vi "Begin.vi"(8 "error in":errorcluster) -> (0 "error out":errorcluster)   [LabVIEW 2019]
doc: "Called before other user functions, this VI is expected to open initial I/O refnums, load in file data, and do all program initialization. Notice that the <B>error out</B> terminal is simply used for data flow. Wiring it to other structures or subVIs ensures that this VI runs first."
uses:
  <vilib>/Rock Robotics/WPI/DriverStation/WPI_DriverStationRobotMode2.ctl
  Subsystems/Drive/Drive_Cluster.ctl
  Subsystems/Drive/Drive_States.ctl
  Subsystems/Intake/Intake_Cluster.ctl
  Subsystems/Intake/Intake_States.ctl
  Subsystems/Turret/Turret_Cluster.ctl
  Subsystems/Turret/Turret_States.ctl
  Subsystems/Magazine/Magazine_Cluster.ctl
  Subsystems/Magazine/Magazine_States.ctl
  Subsystems/Climb/Climb_Cluster.ctl
  Subsystems/Climb/Climb_States.ctl
  Subsystems/Control_Panel/Control_Panel_Cluster.ctl
  Subsystems/Control_Panel/Control_Panel_States.ctl
  <vilib>/Rock Robotics/WPI/Joystick/WPI_JoystickDeviceEnum.ctl
  <vilib>/Rock Robotics/WPI/ThirdParty/REV Robotics/SPARK MAX/Typedef/Spark MAX Control Type.ctl
  Subsystems/Flywheel/Flywheel_Cluster.ctl
  Subsystems/Flywheel/Flywheel_States.ctl
  <vilib>/Rock Robotics/WPI/ThirdParty/Phoenix-LabVIEW/Motor Controller/Controls/CTRE_Phoenix_MotorControl_ControlMode.ctl
  <vilib>/Rock Robotics/WPI/ThirdParty/REV Robotics/SPARK MAX/Typedef/Spark MAX Idle Mode.ctl
  <vilib>/Rock Robotics/WPI/ThirdParty/REV Robotics/SPARK MAX/Typedef/Spark MAX Motor Type.ctl
  <vilib>/Rock Robotics/WPI/ThirdParty/Phoenix-LabVIEW/Motor Controller/Controls/CTRE_Phoenix_MotorControl_SupplyCurrentLimitConfiguration.ctl
  Robot Global Data.vi
  Globals/Drive_Globals.vi
  Globals/Intake_Globals.vi
  Globals/Turret_Globals.vi
  Globals/Magazine_Globals.vi
  Globals/Climb_Globals.vi
  Globals/Control_Panel_Globals.vi
  Globals/Joystick_Globals.vi
  Globals/Flywheel_Globals.vi
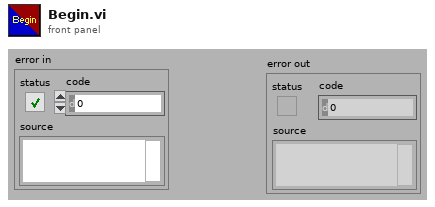
[diagram p1: front panel]
types:
  T1 = typedef "CTRE_Phoenix_MotorControl_SupplyCurrentLimitConfiguration.ctl" = cluster{"Enable?":bool, "Current Limit":dbl, "Threshold Current":dbl, "Threshold Time":dbl}
  T2 = typedef "Spark MAX Idle Mode.ctl" = enum16{"Coast", "Brake"}
  T3 = typedef "Spark MAX Motor Type.ctl" = enum16{"Brushed", "Brushless"}
  T4 = typedef "CTRE_Phoenix_MotorControl_ControlMode.ctl" = u16
  T5 = typedef "Spark MAX Control Type.ctl" = enum16{"Percent VBus", "Voltage", "Velocity", "Position", "Smart Motion", "Current", "Smart Velocity"}
  T6 = cluster{"P Gain":dbl, "I Gain":dbl, "D Gain":dbl, "F Gain":dbl, "I Zone":dbl, "Min Output":dbl, "Max Output":dbl}
  T7 = typedef "Flywheel_Cluster.ctl" = cluster{"Flywheel_Throttle":dbl, "Control_States":T8, "Auto_Speed":bool, "Flywheel_On":bool}
  T8 = typedef "Flywheel_States.ctl" = enum16{"No-Op", "Percent_Voltage", "Speed_Control_Manual", "Speed_Control_Auto"}
  T9 = typedef "WPI_JoystickDeviceEnum.ctl" = enum16{"USB 0", "USB 1", "USB 2", "USB 3", "USB 4", "USB 5"}
  T10 = typedef "Control_Panel_Cluster.ctl" = cluster{"Control_State":T11, "Start_Movement":bool, "Abort":bool, "Rotation_Control?":bool, "Positional_Control? ":bool, "Throttle":dbl}
  T11 = typedef "Control_Panel_States.ctl" = enum16{"No-Op", "Rotational_Control", "Positional_Control", "Manual_Control"}
  T12 = typedef "Climb_Cluster.ctl" = cluster{"Control_State":T13, "Extend_Climber?":bool, "Clamp?":bool, "Balance?":bool, "Transverse_Throttle":dbl, "Elevator_Throttle":dbl, "Control_Panel_Setpoint?":bool, "Auto-Balance":bool, "Pivot_Throttle":dbl}
  T13 = typedef "Climb_States.ctl" = enum16{"No-Op", "Extending", "Clamping", "Balancing", "Manual_Control"}
  T14 = typedef "Magazine_Cluster.ctl" = cluster{"Control_States":T15, "Fire":bool, "Magazine_Throttle":dbl}
  T15 = typedef "Magazine_States.ctl" = enum16{"No-Op", "Loading", "Fire", "Unjam", "Manual"}
  T16 = typedef "Turret_Cluster.ctl" = cluster{"Auto-Target?":bool, "Control_State":T17, "Turret_Spin_Speed":dbl, "Turret_Spin_Speed_Control?":bool}
  T17 = typedef "Turret_States.ctl" = enum16{"Manual_Percent_Voltage", "Manual_Speed_Control", "Auto-Target"}
  T18 = typedef "Intake_Cluster.ctl" = cluster{"Control_State":T19, "Intake_On":bool, "Intake_Extended":bool, "Intake_Throttle":dbl}
  T19 = typedef "Intake_States.ctl" = enum16{"Manual_Control"}
  T20 = typedef "Drive_Cluster.ctl" = cluster{"Control_State":T21, "Angular_Throttle":dbl, "Linear_Throttle":dbl, "Torque_Changing":bool}
  T21 = typedef "Drive_States.ctl" = enum16{"Percent_Voltage_Control", "Speed_Control"}
  T22 = typedef "WPI_DriverStationRobotMode2.ctl" = enum16{"Autonomous Disabled", "Autonomous Enabled", "Teleop Disabled", "Teleop Enabled", "Disconnected", "Finish", "Test Disabled", "Test Enabled", "Emergency Stopped"}
  T23 = typedef "WPI_JoystickDevRef.ctl" = cluster{"Device":T9}
  T24 = typedef "WPI_MotorControlDeviceRef.ctl" = cluster{"DeviceStatus":errorcluster, "Type":T25, "PWM":cluster{"PWM Channel":T26, "DeadBand":T27}, "CAN":cluster{"Device Number":u8, "SetOutput VI Ref":variant, "GetOutput VI Ref":variant, "Enable VI Ref":variant, "Disable VI Ref":variant, "Data":variant}, "Invert":bool, "DIO PWM":cluster{"PWM \"Enable\" Channel":T26, "DIOChannel":T28, "PWM Rate":dbl}}
  T25 = typedef "WPI_MotorControlType.ctl" = enum16{"PWM", "CAN", "DIO PWM"}
  T26 = typedef "FPGA_DIOPWMChannel.ctl" = enum8{"PWM 0", "PWM 1", "PWM 2", "PWM 3", "PWM 4", "PWM 5", "PWM 6", "PWM 7", "PWM 8", "PWM 9", "PWM MXP 0", "PWM MXP 1", "PWM MXP 2", "PWM MXP 3", "PWM MXP 4", "PWM MXP 5", "PWM MXP 6", "PWM MXP 7", "PWM MXP 8", "PWM MXP 9", "Invalid"}
  T27 = typedef "WPI_PWMDeadband.ctl" = cluster{"Name":string, "maxPositivePwm":i32, "minPositivePwm":i32, "centerPwm":i32, "maxNegativePwm":i32, "minNegativePwm":i32, "angularRange":u16}
  T28 = typedef "FPGA_DIOChannel.ctl" = enum8{"DIO 0", "DIO 1", "DIO 2", "DIO 3", "DIO 4", "DIO 5", "DIO 6", "DIO 7", "DIO 8", "DIO 9", "DIO MXP 0", "DIO MXP 1", "DIO MXP 2", "DIO MXP 3", "DIO MXP 4", "DIO MXP 5", "DIO MXP 6", "DIO MXP 7", "DIO MXP 8", "DIO MXP 9", "DIO MXP 10", "DIO MXP 11", "DIO MXP 12", "DIO MXP 13", "DIO MXP 14", "DIO MXP 15", "SPI Port CS1", "SPI Port CS2", "SPI Port CS3", "SPI Port MISO", "SPI Port MOSI", "Invalid"}
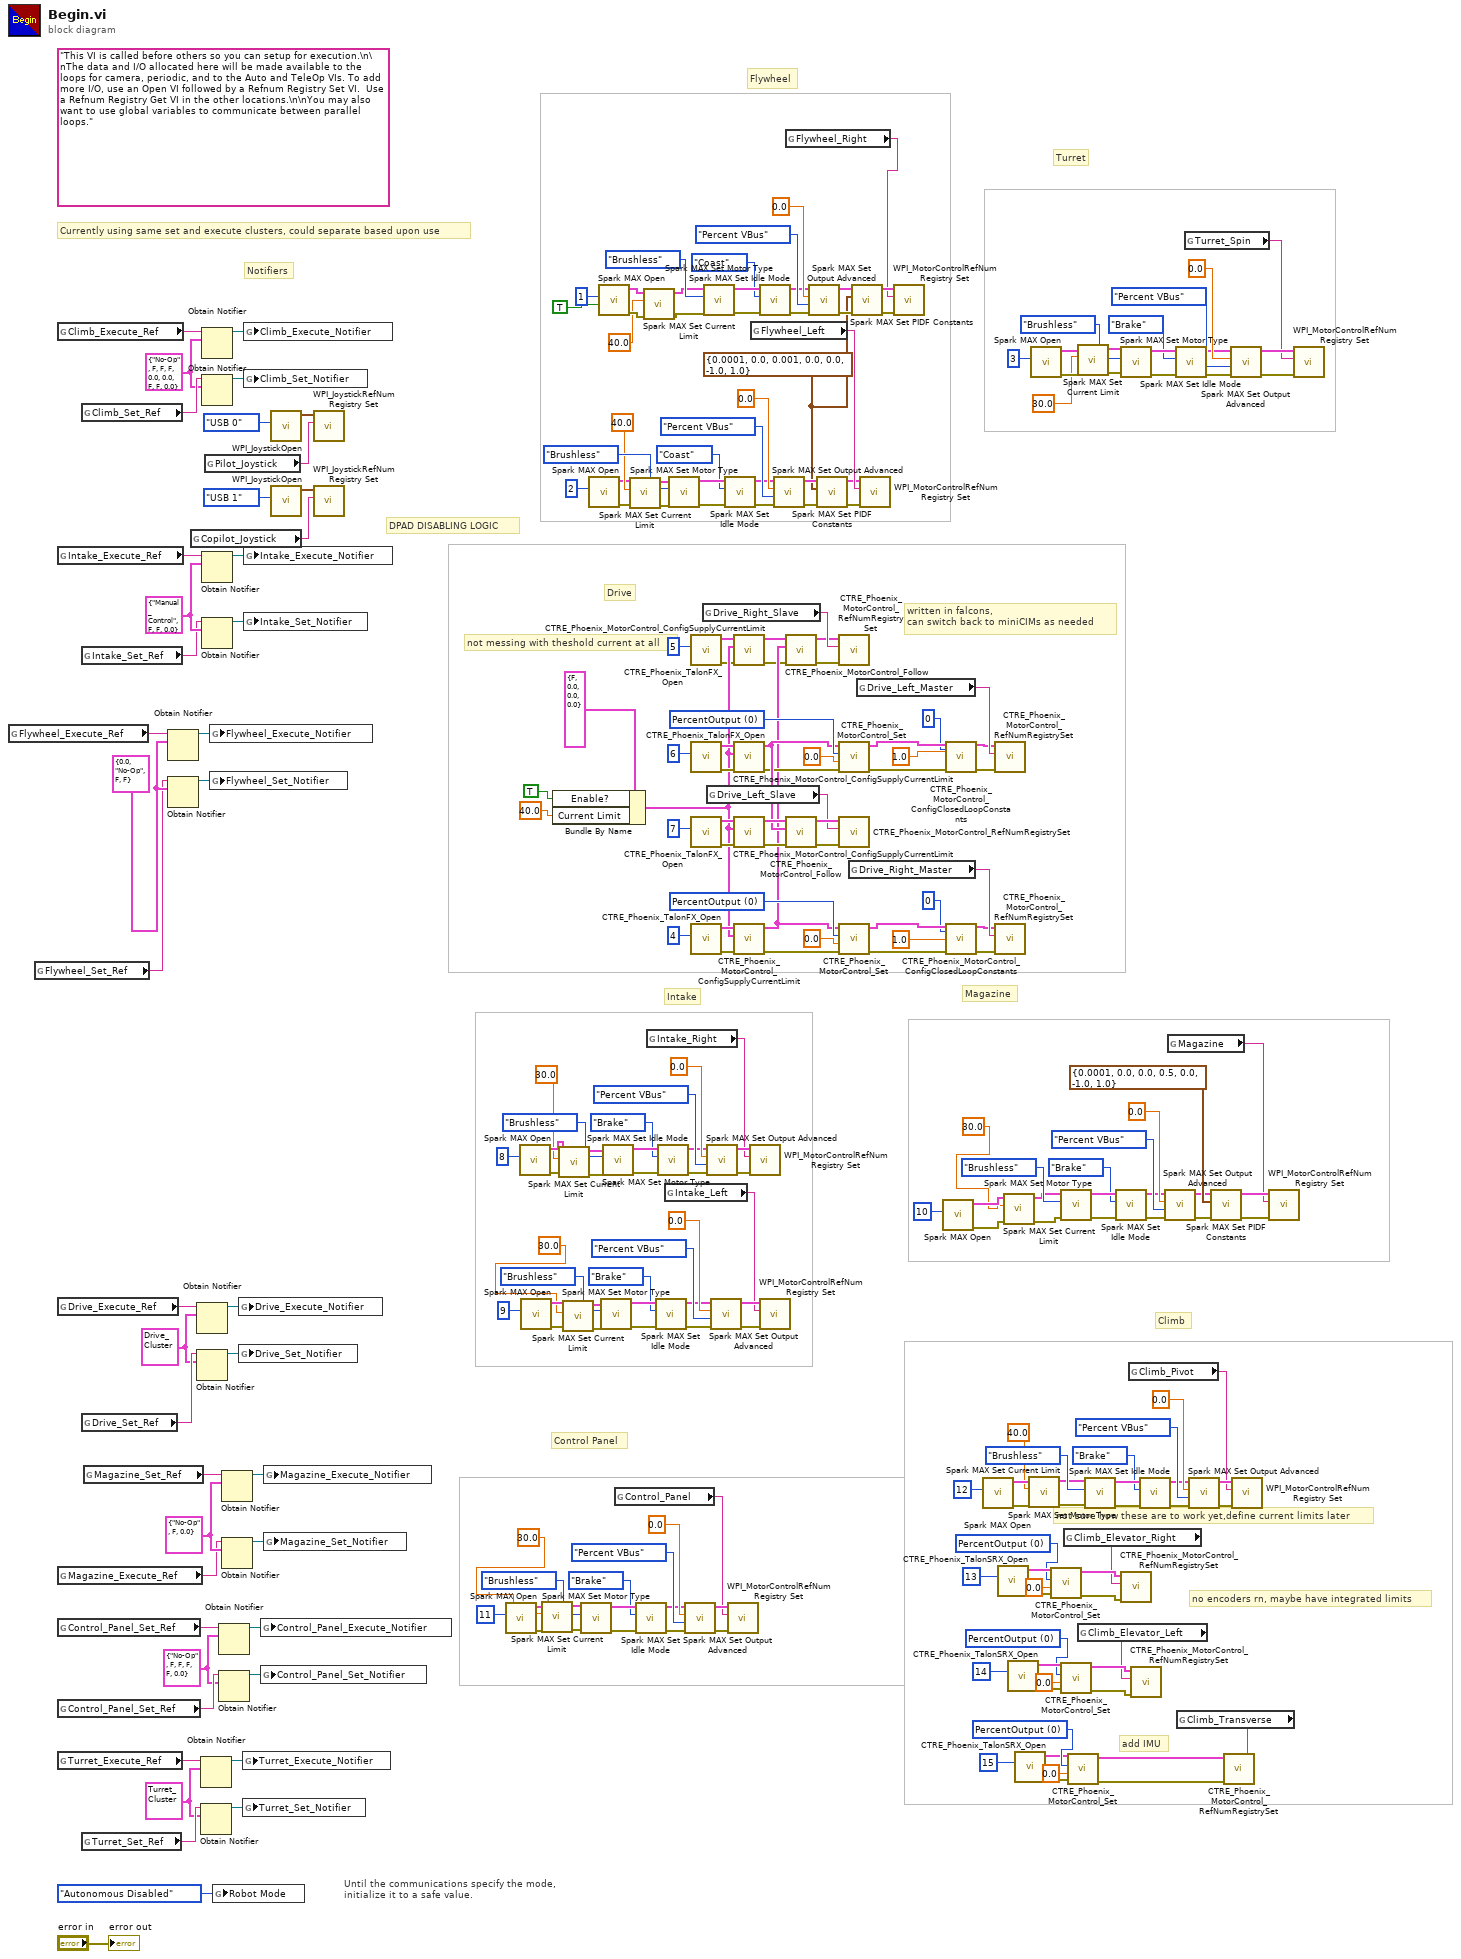
[diagram p0: block diagram]
diagram:
  w119 = T4 0 items=["PercentOutput"=0, "Position"=1, "Velocity"=2, "Current"=3, "Follower"=5, "MotionProfile"=6, "MotionMagic"=7, "MotionProfileArc"=10, "Disabled"=15] ("Control Mode")
  w126 = T4 0 items=["PercentOutput"=0, "Position"=1, "Velocity"=2, "Current"=3, "Follower"=5, "MotionProfile"=6, "MotionMagic"=7, "MotionProfileArc"=10, "Disabled"=15] ("Control Mode")
  w135 = T4 0 items=["PercentOutput"=0, "Position"=1, "Velocity"=2, "Current"=3, "Follower"=5, "MotionProfile"=6, "MotionMagic"=7, "MotionProfileArc"=10, "Disabled"=15] ("Control Mode")
  w168 = T7 {"Flywheel_Throttle"=0.0, "Control_States"=enum."No-Op", "Auto_Speed"=FALSE, "Flywheel_On"=FALSE}
  w1 = T6 {"P Gain"=0.0001, "I Gain"=0.0, "D Gain"=0.001, "F Gain"=0.0, "I Zone"=0.0, "Min Output"=-1.0, "Max Output"=1.0} ("PID Constants")
  w207 = T4 0 items=["PercentOutput"=0, "Position"=1, "Velocity"=2, "Current"=3, "Follower"=5, "MotionProfile"=6, "MotionMagic"=7, "MotionProfileArc"=10, "Disabled"=15] ("Control Mode")
  w217 = T4 0 items=["PercentOutput"=0, "Position"=1, "Velocity"=2, "Current"=3, "Follower"=5, "MotionProfile"=6, "MotionMagic"=7, "MotionProfileArc"=10, "Disabled"=15] ("Control Mode")
  w241 = T10 {"Control_State"=enum."No-Op", "Start_Movement"=FALSE, "Abort"=FALSE, "Rotation_Control?"=FALSE, "Positional_Control? "=FALSE, "Throttle"=0.0}
  w245 = T12 {"Control_State"=enum."No-Op", "Extend_Climber?"=FALSE, "Clamp?"=FALSE, "Balance?"=FALSE, "Transverse_Throttle"=0.0, "Elevator_Throttle"=0.0, "Control_Panel_Setpoint?"=FALSE, "Auto-Balance"=FALSE, "Pivot_Throttle"=0.0}
  w249 = T14 {"Control_States"=enum."No-Op", "Fire"=FALSE, "Magazine_Throttle"=0.0}
  w250 = T16 {"Auto-Target?"=FALSE, "Control_State"=enum."Manual_Percent_Voltage", "Turret_Spin_Speed"=0.0, "Turret_Spin_Speed_Control?"=FALSE}
  w255 = T18 {"Control_State"=enum."Manual_Control", "Intake_On"=FALSE, "Intake_Extended"=FALSE, "Intake_Throttle"=0.0}
  w256 = T20 {"Control_State"=enum."Percent_Voltage_Control", "Angular_Throttle"=0.0, "Linear_Throttle"=0.0, "Torque_Changing"=FALSE}
  (unwired) "This VI is called before others so you can setup for execution.\n\nThe data and I/O allocated here will be made available to the loops for camera, periodic, and to the Auto and TeleOp VIs. To add more I/O, use an Open VI followed by a Refnum Registry Set VI.  Use a Refnum Registry Get VI in the other locations.\n\nYou may also want to use global variables to communicate between parallel loops."
  # "not sure how these are to work yet,define current limits later"
  # "not messing with theshold current at all"
  # "add IMU"
  # "no encoders rn, maybe have integrated limits"
  # "Climb"
  # "Control Panel"
  # "Magazine"
  # "Intake"
  # "written in falcons, \ncan switch back to miniCIMs as needed"
  # "Drive"
  # "Turret"
  # "Flywheel"
  # "DPAD DISABLING LOGIC"
  # "Notifiers"
  # "Currently using same set and execute clusters, could separate based upon use"
  # "Until the communications specify the mode,\ninitialize it to a safe value."
  n1 = global read "Flywheel_Globals.vi" "Flywheel_Execute_Ref"() -> (w167:string)
  n2 = global read "Flywheel_Globals.vi" "Flywheel_Set_Ref"() -> (w166:string)
  n3 = global read "Climb_Globals.vi" "Climb_Execute_Ref"() -> (w244:string)
  n4 = global read "Intake_Globals.vi" "Intake_Execute_Ref"() -> (w254:string)
  n5 = global read "Drive_Globals.vi" "Drive_Execute_Ref"() -> (w257:string)
  n6 = global read "Magazine_Globals.vi" "Magazine_Execute_Ref"() -> (w248:string)
  n7 = global read "Control_Panel_Globals.vi" "Control_Panel_Set_Ref"() -> (w243:string)
  n8 = global read "Control_Panel_Globals.vi" "Control_Panel_Set_Ref"() -> (w242:string)
  n9 = global read "Turret_Globals.vi" "Turret_Execute_Ref"() -> (w252:string)
  n10 = global read "Climb_Globals.vi" "Climb_Set_Ref"() -> (w246:string)
  n11 = global read "Intake_Globals.vi" "Intake_Set_Ref"() -> (w253:string)
  n12 = global read "Drive_Globals.vi" "Drive_Set_Ref"() -> (w258:string)
  n13 = global read "Turret_Globals.vi" "Turret_Set_Ref"() -> (w251:string)
  n14 = global read "Magazine_Globals.vi" "Magazine_Set_Ref"() -> (w247:string)
  n15 = Obtain Notifier(name (unnamed)=w167, notification data type=w168) -> (notifier out=w164:refnum<notifier>)  [unwired: 2 in, 2 out]
  n16 = Obtain Notifier(name (unnamed)=w166, notification data type=w168) -> (notifier out=w165:refnum<notifier>)  [unwired: 2 in, 2 out]
  n17 = global read "Joystick_Globals.vi" "Copilot_Joystick"() -> (w223:string)
  n18 = Obtain Notifier(name (unnamed)=w257, notification data type=w256) -> (notifier out=w235:refnum<notifier>)  [unwired: 2 in, 2 out]
  n19 = Obtain Notifier(name (unnamed)=w258, notification data type=w256) -> (notifier out=w236:refnum<notifier>)  [unwired: 2 in, 2 out]
  n20 = Obtain Notifier(name (unnamed)=w252, notification data type=w250) -> (notifier out=w229:refnum<notifier>)  [unwired: 2 in, 2 out]
  n21 = Obtain Notifier(name (unnamed)=w251, notification data type=w250) -> (notifier out=w230:refnum<notifier>)  [unwired: 2 in, 2 out]
  n22 = Obtain Notifier(name (unnamed)=w244, notification data type=w245) -> (notifier out=w239:refnum<notifier>)  [unwired: 2 in, 2 out]
  n23 = Obtain Notifier(name (unnamed)=w246, notification data type=w245) -> (notifier out=w240:refnum<notifier>)  [unwired: 2 in, 2 out]
  n24 = Obtain Notifier(name (unnamed)=w254, notification data type=w255) -> (notifier out=w237:refnum<notifier>)  [unwired: 2 in, 2 out]
  n25 = Obtain Notifier(name (unnamed)=w253, notification data type=w255) -> (notifier out=w238:refnum<notifier>)  [unwired: 2 in, 2 out]
  n26 = global read "Joystick_Globals.vi" "Pilot_Joystick"() -> (w224:string)
  n27 = global write "Flywheel_Globals.vi" "Flywheel_Execute_Notifier"(w164) -> ()
  n28 = global write "Flywheel_Globals.vi" "Flywheel_Set_Notifier"(w165) -> ()
  n29 = global write "Robot Global Data.vi" "Robot Mode"(WPI_DriverStationRobotMode2."Autonomous Disabled" ("Robot Mode")) -> ()
  n30 = Obtain Notifier(name (unnamed)=w243, notification data type=w241) -> (notifier out=w231:refnum<notifier>)  [unwired: 2 in, 2 out]
  n31 = Obtain Notifier(name (unnamed)=w242, notification data type=w241) -> (notifier out=w232:refnum<notifier>)  [unwired: 2 in, 2 out]
  n32 = Obtain Notifier(name (unnamed)=w247, notification data type=w249) -> (notifier out=w233:refnum<notifier>)  [unwired: 2 in, 2 out]
  n33 = Obtain Notifier(name (unnamed)=w248, notification data type=w249) -> (notifier out=w234:refnum<notifier>)  [unwired: 2 in, 2 out]
  n34 = global write "Drive_Globals.vi" "Drive_Execute_Notifier"(w235) -> ()
  n35 = global write "Drive_Globals.vi" "Drive_Set_Notifier"(w236) -> ()
  n36 = global write "Turret_Globals.vi" "Turret_Execute_Notifier"(w229) -> ()
  n37 = global write "Turret_Globals.vi" "Turret_Set_Notifier"(w230) -> ()
  n38 = global write "Climb_Globals.vi" "Climb_Execute_Notifier"(w239) -> ()
  n39 = global write "Climb_Globals.vi" "Climb_Set_Notifier"(w240) -> ()
  n40 = global write "Intake_Globals.vi" "Intake_Execute_Notifier"(w237) -> ()
  n41 = global write "Intake_Globals.vi" "Intake_Set_Notifier"(w238) -> ()
  n42 = global write "Control_Panel_Globals.vi" "Control_Panel_Execute_Notifier"(w231) -> ()
  n43 = global write "Control_Panel_Globals.vi" "Control_Panel_Set_Notifier"(w232) -> ()
  n44 = global write "Magazine_Globals.vi" "Magazine_Execute_Notifier"(w233) -> ()
  n45 = global write "Magazine_Globals.vi" "Magazine_Set_Notifier"(w234) -> ()
  n46 = call <vilib>:"WPI_JoystickOpen.vi"("JoystickDevice"=WPI_JoystickDeviceEnum."USB 0") -> ("JoystickDevRef"=w228:T23)  [unwired: 10 in]
  n47 = call <vilib>:"WPI_JoystickOpen.vi"("JoystickDevice"=WPI_JoystickDeviceEnum."USB 1") -> ("JoystickDevRef"=w227:T23)  [unwired: 10 in]
  n48 = call <vilib>:"WPI_JoystickRefNum Registry Set.vi"("refnum name"=w224, "JoystickDevRef"=w228) -> ()  [unwired: 8 in, 2 out]
  n49 = call <vilib>:"WPI_JoystickRefNum Registry Set.vi"("refnum name"=w223, "JoystickDevRef"=w227) -> ()  [unwired: 8 in, 2 out]
  n50 = call <vilib>:"Spark MAX Open.vi"("Device Number"=u8 11) -> ("error out"=w26:errorcluster, "MotorControlDeviceRef"=w25:T24)  [unwired: 9 in]
  n51 = call <vilib>:"Spark MAX Open.vi"("Device Number"=u8 8) -> ("error out"=w41:errorcluster, "MotorControlDeviceRef"=w40:T24)  [unwired: 9 in]
  n52 = call <vilib>:"Spark MAX Open.vi"("Device Number"=u8 9) -> ("error out"=w33:errorcluster, "MotorControlDeviceRef"=w34:T24)  [unwired: 9 in]
  n53 = call <vilib>:"Spark MAX Set Current Limit.vi"("error in (no error)"=w26, "Current Limit A (100)"=sgl 30.0, "MotorControlDeviceRef in"=w25) -> ("error out"=w23:errorcluster, "MotorControlDeviceRef out"=w24:T24)  [unwired: 7 in]
  n54 = Bundle By Name(cluster=T1 {"Enable?"=FALSE, "Current Limit"=0.0, "Threshold Current"=0.0, "Threshold Time"=0.0} ("Supply Current Limit Configuration"), "Enable?"=TRUE, "Current Limit"=40.0) -> (w5:T1)
  n55 = call <vilib>:"Spark MAX Set Current Limit.vi"("error in (no error)"=w41, "Current Limit A (100)"=sgl 30.0, "MotorControlDeviceRef in"=w40) -> ("error out"=w38:errorcluster, "MotorControlDeviceRef out"=w39:T24)  [unwired: 7 in]
  n56 = call <vilib>:"Spark MAX Set Current Limit.vi"("error in (no error)"=w33, "Current Limit A (100)"=sgl 30.0, "MotorControlDeviceRef in"=w34) -> ("error out"=w36:errorcluster, "MotorControlDeviceRef out"=w35:T24)  [unwired: 7 in]
  n57 = call <vilib>:"Spark MAX Set Motor Type.vi"("error in (no error)"=w23, "Motor Type"=Spark_MAX_Motor_Type."Brushless", "MotorControlDevRef"=w24) -> ("error out"=w68:errorcluster, "MotorControlDeviceRef"=w65:T24)  [unwired: 7 in]
  n58 = call <vilib>:"Spark MAX Open.vi"("Device Number"=u8 2) -> ("error out"=w50:errorcluster, "MotorControlDeviceRef"=w49:T24)  [unwired: 9 in]
  n59 = call <vilib>:"Spark MAX Open.vi"("Invert"=TRUE, "Device Number"=u8 1) -> ("error out"=w56:errorcluster, "MotorControlDeviceRef"=w55:T24)  [unwired: 8 in]
  n60 = call <vilib>:"Spark MAX Set Motor Type.vi"("error in (no error)"=w36, "Motor Type"=Spark_MAX_Motor_Type."Brushless", "MotorControlDevRef"=w35) -> ("error out"=w87:errorcluster, "MotorControlDeviceRef"=w84:T24)  [unwired: 7 in]
  n61 = call <vilib>:"Spark MAX Set Motor Type.vi"("error in (no error)"=w38, "Motor Type"=Spark_MAX_Motor_Type."Brushless", "MotorControlDevRef"=w39) -> ("error out"=w93:errorcluster, "MotorControlDeviceRef"=w92:T24)  [unwired: 7 in]
  n62 = global read "Control_Panel_Globals.vi" "Control_Panel"() -> (w144:string)
  n63 = call <vilib>:"Spark MAX Set Current Limit.vi"("error in (no error)"=w50, "Current Limit A (100)"=sgl 40.0, "MotorControlDeviceRef in"=w49) -> ("error out"=w47:errorcluster, "MotorControlDeviceRef out"=w48:T24)  [unwired: 7 in]
  n64 = call <vilib>:"Spark MAX Set Idle Mode.vi"("error in (no error)"=w68, "Idle Mode"=Spark_MAX_Idle_Mode."Brake", "MotorControlDeviceRef in"=w65) -> ("error out"=w67:errorcluster, "MotorControlDeviceRef out"=w66:T24)  [unwired: 7 in]
  n65 = call <vilib>:"Spark MAX Set Current Limit.vi"("error in (no error)"=w56, "Current Limit A (100)"=sgl 40.0, "MotorControlDeviceRef in"=w55) -> ("error out"=w54:errorcluster, "MotorControlDeviceRef out"=w53:T24)  [unwired: 7 in]
  n66 = global read "Intake_Globals.vi" "Intake_Right"() -> (w171:string)
  n67 = call <vilib>:"Spark MAX Set Idle Mode.vi"("error in (no error)"=w87, "Idle Mode"=Spark_MAX_Idle_Mode."Brake", "MotorControlDeviceRef in"=w84) -> ("error out"=w86:errorcluster, "MotorControlDeviceRef out"=w85:T24)  [unwired: 7 in]
  n68 = call <vilib>:"Spark MAX Set Idle Mode.vi"("error in (no error)"=w93, "Idle Mode"=Spark_MAX_Idle_Mode."Brake", "MotorControlDeviceRef in"=w92) -> ("error out"=w90:errorcluster, "MotorControlDeviceRef out"=w91:T24)  [unwired: 7 in]
  n69 = global read "Intake_Globals.vi" "Intake_Left"() -> (w170:string)
  n70 = call <vilib>:"Spark MAX Set Motor Type.vi"("error in (no error)"=w47, "Motor Type"=Spark_MAX_Motor_Type."Brushless", "MotorControlDevRef"=w48) -> ("error out"=w106:errorcluster, "MotorControlDeviceRef"=w105:T24)  [unwired: 7 in]
  n71 = call <vilib>:"Spark MAX Set Output Advanced.vi"("error in (no error)"=w67, "Control Mode"=Spark_MAX_Control_Type."Percent VBus", "Setpoint"=0.0, "MotorControlDevRef"=w66) -> ("error out"=w69:errorcluster, "MotorControlDevRef"=w147:T24)  [unwired: 6 in]
  n72 = call <vilib>:"CTRE_Phoenix_TalonFX_Open.vi"("Device Number"=u8 5) -> ("error out"=w4:errorcluster, "CAN Talon SRX Ref"=w3:T24)  [unwired: 9 in]
  n73 = call <vilib>:"CTRE_Phoenix_TalonFX_Open.vi"("Device Number"=u8 6) -> ("error out"=w13:errorcluster, "CAN Talon SRX Ref"=w12:T24)  [unwired: 9 in]
  n74 = call <vilib>:"CTRE_Phoenix_TalonFX_Open.vi"("Device Number"=u8 7) -> ("error out"=w16:errorcluster, "CAN Talon SRX Ref"=w17:T24)  [unwired: 9 in]
  n75 = call <vilib>:"CTRE_Phoenix_TalonFX_Open.vi"("Device Number"=u8 4) -> ("error out"=w8:errorcluster, "CAN Talon SRX Ref"=w9:T24)  [unwired: 9 in]
  n76 = global read "Drive_Globals.vi" "Drive_Right_Slave"() -> (w214:string)
  n77 = call <vilib>:"Spark MAX Set Motor Type.vi"("error in (no error)"=w54, "Motor Type"=Spark_MAX_Motor_Type."Brushless", "MotorControlDevRef"=w53) -> ("error out"=w111:errorcluster, "MotorControlDeviceRef"=w112:T24)  [unwired: 7 in]
  n78 = global read "Drive_Globals.vi" "Drive_Left_Slave"() -> (w206:string)
  n79 = call <vilib>:"Spark MAX Set Output Advanced.vi"("error in (no error)"=w90, "Control Mode"=Spark_MAX_Control_Type."Percent VBus", "Setpoint"=0.0, "MotorControlDevRef"=w91) -> ("error out"=w178:errorcluster, "MotorControlDevRef"=w179:T24)  [unwired: 6 in]
  n80 = call <vilib>:"Spark MAX Set Output Advanced.vi"("error in (no error)"=w86, "Control Mode"=Spark_MAX_Control_Type."Percent VBus", "Setpoint"=0.0, "MotorControlDevRef"=w85) -> ("error out"=w169:errorcluster, "MotorControlDevRef"=w173:T24)  [unwired: 6 in]
  n81 = call <vilib>:"Spark MAX Set Idle Mode.vi"("error in (no error)"=w106, "Idle Mode"=Spark_MAX_Idle_Mode."Coast", "MotorControlDeviceRef in"=w105) -> ("error out"=w104:errorcluster, "MotorControlDeviceRef out"=w103:T24)  [unwired: 7 in]
  n82 = call <vilib>:"WPI_MotorControlRefNum Registry Set.vi"("error in (no error)"=w69, "refnum name"=w144, "MotorControlDevRef"=w147) -> ()  [unwired: 7 in, 2 out]
  n83 = call <vilib>:"CTRE_Phoenix_MotorControl_ConfigSupplyCurrentLimit.vi"("error in (no error)"=w4, "Supply Current Limit Configuration"=w5, "PhoenixMotorControlDevRef"=w3) -> ("error out"=w7:errorcluster, "PhoenixMotorControlDevRef"=w6:T24)  [unwired: 7 in]
  n84 = call <vilib>:"CTRE_Phoenix_MotorControl_ConfigSupplyCurrentLimit.vi"("error in (no error)"=w13, "Supply Current Limit Configuration"=w5, "PhoenixMotorControlDevRef"=w12) -> ("error out"=w14:errorcluster, "PhoenixMotorControlDevRef"=w15:T24)  [unwired: 7 in]
  n85 = call <vilib>:"CTRE_Phoenix_MotorControl_ConfigSupplyCurrentLimit.vi"("error in (no error)"=w16, "Supply Current Limit Configuration"=w5, "PhoenixMotorControlDevRef"=w17) -> ("error out"=w21:errorcluster, "PhoenixMotorControlDevRef"=w20:T24)  [unwired: 7 in]
  n86 = call <vilib>:"CTRE_Phoenix_MotorControl_ConfigSupplyCurrentLimit.vi"("error in (no error)"=w8, "Supply Current Limit Configuration"=w5, "PhoenixMotorControlDevRef"=w9) -> ("error out"=w11:errorcluster, "PhoenixMotorControlDevRef"=w10:T24)  [unwired: 7 in]
  n87 = call <vilib>:"WPI_MotorControlRefNum Registry Set.vi"("error in (no error)"=w178, "refnum name"=w171, "MotorControlDevRef"=w179) -> ()  [unwired: 7 in, 2 out]
  n88 = global read "Flywheel_Globals.vi" "Flywheel_Left"() -> (w221:string)
  n89 = call <vilib>:"Spark MAX Set Idle Mode.vi"("error in (no error)"=w111, "Idle Mode"=Spark_MAX_Idle_Mode."Coast", "MotorControlDeviceRef in"=w112) -> ("error out"=w107:errorcluster, "MotorControlDeviceRef out"=w108:T24)  [unwired: 7 in]
  n90 = call <vilib>:"WPI_MotorControlRefNum Registry Set.vi"("error in (no error)"=w169, "refnum name"=w170, "MotorControlDevRef"=w173) -> ()  [unwired: 7 in, 2 out]
  n91 = call <vilib>:"Spark MAX Set Output Advanced.vi"("error in (no error)"=w104, "Control Mode"=Spark_MAX_Control_Type."Percent VBus", "Setpoint"=0.0, "MotorControlDevRef"=w103) -> ("error out"=w190:errorcluster, "MotorControlDevRef"=w189:T24)  [unwired: 6 in]
  n92 = global read "Flywheel_Globals.vi" "Flywheel_Right"() -> (w183:string)
  n93 = call <vilib>:"CTRE_Phoenix_MotorControl_Follow.vi"("error in (no error)"=w7, "Master Controller to Follow"=w10, "PhoenixMotorControlDevRef"=w6) -> ("error out"=w212:errorcluster, "PhoenixMotorControlDevRef"=w213:T24)  [unwired: 7 in]
  n94 = call <vilib>:"CTRE_Phoenix_MotorControl_Follow.vi"("error in (no error)"=w21, "Master Controller to Follow"=w15, "PhoenixMotorControlDevRef"=w20) -> ("error out"=w211:errorcluster, "PhoenixMotorControlDevRef"=w210:T24)  [unwired: 7 in]
  n95 = call <vilib>:"Spark MAX Set Output Advanced.vi"("error in (no error)"=w107, "Control Mode"=Spark_MAX_Control_Type."Percent VBus", "Setpoint"=0.0, "MotorControlDevRef"=w108) -> ("error out"=w154:errorcluster, "MotorControlDevRef"=w185:T24)  [unwired: 6 in]
  n96 = call <vilib>:"Spark MAX Set PIDF Constants.vi"("error in"=w190, "PID Constants"=w1, "MotorControlDeviceRef"=w189) -> ("error out"=w188:errorcluster, "MotorControlDeviceRef"=w187:T24)  [unwired: 7 in]
  n97 = call <vilib>:"CTRE_Phoenix_MotorControl_RefNumRegistrySet.vi"("error in (no error)"=w212, "refnum name"=w214, "PhoenixMotorControlDevRef"=w213) -> ()  [unwired: 7 in, 2 out]
  n98 = call <vilib>:"CTRE_Phoenix_MotorControl_Set.vi"("error in (no error)"=w14, "Output"=0.0, "Control Mode"=w207, "PhoenixMotorControlDevRef"=w15) -> ("error out"=w200:errorcluster, "PhoenixMotorControlDevRef"=w201:T24)  [unwired: 6 in]
  n99 = call <vilib>:"CTRE_Phoenix_MotorControl_RefNumRegistrySet.vi"("error in (no error)"=w211, "refnum name"=w206, "PhoenixMotorControlDevRef"=w210) -> ()  [unwired: 7 in, 2 out]
  n100 = call <vilib>:"CTRE_Phoenix_MotorControl_Set.vi"("error in (no error)"=w11, "Output"=0.0, "Control Mode"=w217, "PhoenixMotorControlDevRef"=w10) -> ("error out"=w198:errorcluster, "PhoenixMotorControlDevRef"=w199:T24)  [unwired: 6 in]
  n101 = global read "Drive_Globals.vi" "Drive_Right_Master"() -> (w215:string)
  n102 = call <vilib>:"Spark MAX Set PIDF Constants.vi"("error in"=w154, "PID Constants"=w1, "MotorControlDeviceRef"=w185) -> ("error out"=w153:errorcluster, "MotorControlDeviceRef"=w186:T24)  [unwired: 7 in]
  n103 = global read "Drive_Globals.vi" "Drive_Left_Master"() -> (w209:string)
  n104 = call <vilib>:"WPI_MotorControlRefNum Registry Set.vi"("error in (no error)"=w188, "refnum name"=w221, "MotorControlDevRef"=w187) -> ()  [unwired: 7 in, 2 out]
  n105 = call <vilib>:"WPI_MotorControlRefNum Registry Set.vi"("error in (no error)"=w153, "refnum name"=w183, "MotorControlDevRef"=w186) -> ()  [unwired: 7 in, 2 out]
  n106 = call <vilib>:"Spark MAX Open.vi"("Device Number"=u8 10) -> ("error out"=w58:errorcluster, "MotorControlDeviceRef"=w59:T24)  [unwired: 9 in]
  n107 = call <vilib>:"CTRE_Phoenix_MotorControl_ConfigClosedLoopConstants.vi"("PhoenixMotorControlDevRef"=w201, "slotIdx"=0, "P"=1.0, "error in (no error)"=w200) -> ("PhoenixMotorControlDevRef"=w114:T24, "error out"=w113:errorcluster)  [unwired: 10 in]
  n108 = call <vilib>:"CTRE_Phoenix_MotorControl_ConfigClosedLoopConstants.vi"("PhoenixMotorControlDevRef"=w199, "slotIdx"=0, "I"=1.0 ("P"), "error in (no error)"=w198) -> ("PhoenixMotorControlDevRef"=w196:T24, "error out"=w197:errorcluster)  [unwired: 10 in]
  n109 = call <vilib>:"Spark MAX Open.vi"("Device Number"=u8 12) -> ("error out"=w31:errorcluster, "MotorControlDeviceRef"=w30:T24)  [unwired: 9 in]
  n110 = call <vilib>:"CTRE_Phoenix_MotorControl_RefNumRegistrySet.vi"("error in (no error)"=w113, "refnum name"=w209, "PhoenixMotorControlDevRef"=w114) -> ()  [unwired: 7 in, 2 out]
  n111 = call <vilib>:"CTRE_Phoenix_MotorControl_RefNumRegistrySet.vi"("error in (no error)"=w197, "refnum name"=w215, "PhoenixMotorControlDevRef"=w196) -> ()  [unwired: 7 in, 2 out]
  n112 = call <vilib>:"CTRE_Phoenix_TalonSRX_Open.vi"("Device Number"=u8 13) -> ("error out"=w138:errorcluster, "CAN Talon SRX Ref"=w137:T24)  [unwired: 9 in]
  n113 = call <vilib>:"Spark MAX Set Current Limit.vi"("error in (no error)"=w58, "Current Limit A (100)"=sgl 30.0, "MotorControlDeviceRef in"=w59) -> ("error out"=w61:errorcluster, "MotorControlDeviceRef out"=w60:T24)  [unwired: 7 in]
  n114 = call <vilib>:"CTRE_Phoenix_TalonSRX_Open.vi"("Device Number"=u8 14) -> ("error out"=w122:errorcluster, "CAN Talon SRX Ref"=w121:T24)  [unwired: 9 in]
  n115 = call <vilib>:"CTRE_Phoenix_TalonSRX_Open.vi"("Device Number"=u8 15) -> ("error out"=w123:errorcluster, "CAN Talon SRX Ref"=w124:T24)  [unwired: 9 in]
  n116 = call <vilib>:"Spark MAX Set Current Limit.vi"("error in (no error)"=w31, "Current Limit A (100)"=sgl 40.0, "MotorControlDeviceRef in"=w30) -> ("error out"=w28:errorcluster, "MotorControlDeviceRef out"=w29:T24)  [unwired: 7 in]
  n117 = call <vilib>:"Spark MAX Open.vi"("Device Number"=u8 3) -> ("error out"=w46:errorcluster, "MotorControlDeviceRef"=w45:T24)  [unwired: 9 in]
  n118 = call <vilib>:"CTRE_Phoenix_MotorControl_Set.vi"("error in (no error)"=w138, "Output"=0.0, "Control Mode"=w135, "PhoenixMotorControlDevRef"=w137) -> ("error out"=w133:errorcluster, "PhoenixMotorControlDevRef"=w132:T24)  [unwired: 6 in]
  n119 = call <vilib>:"Spark MAX Set Motor Type.vi"("error in (no error)"=w61, "Motor Type"=Spark_MAX_Motor_Type."Brushless", "MotorControlDevRef"=w60) -> ("error out"=w81:errorcluster, "MotorControlDeviceRef"=w80:T24)  [unwired: 7 in]
  n120 = call <vilib>:"CTRE_Phoenix_MotorControl_Set.vi"("error in (no error)"=w122, "Output"=0.0, "Control Mode"=w119, "PhoenixMotorControlDevRef"=w121) -> ("error out"=w117:errorcluster, "PhoenixMotorControlDevRef"=w116:T24)  [unwired: 6 in]
  n121 = global read "Climb_Globals.vi" "Climb_Elevator_Right"() -> (w131:string)
  n122 = call <vilib>:"CTRE_Phoenix_MotorControl_Set.vi"("error in (no error)"=w123, "Output"=0.0, "Control Mode"=w126, "PhoenixMotorControlDevRef"=w124) -> ("error out"=w128:errorcluster, "PhoenixMotorControlDevRef"=w129:T24)  [unwired: 6 in]
  n123 = call <vilib>:"Spark MAX Set Current Limit.vi"("error in (no error)"=w46, "Current Limit A (100)"=sgl 30.0, "MotorControlDeviceRef in"=w45) -> ("error out"=w43:errorcluster, "MotorControlDeviceRef out"=w44:T24)  [unwired: 7 in]
  n124 = global read "Climb_Globals.vi" "Climb_Elevator_Left"() -> (w115:string)
  n125 = call <vilib>:"Spark MAX Set Motor Type.vi"("error in (no error)"=w28, "Motor Type"=Spark_MAX_Motor_Type."Brushless", "MotorControlDevRef"=w29) -> ("error out"=w75:errorcluster, "MotorControlDeviceRef"=w72:T24)  [unwired: 7 in]
  n126 = call <vilib>:"Spark MAX Set Idle Mode.vi"("error in (no error)"=w81, "Idle Mode"=Spark_MAX_Idle_Mode."Brake", "MotorControlDeviceRef in"=w80) -> ("error out"=w79:errorcluster, "MotorControlDeviceRef out"=w78:T24)  [unwired: 7 in]
  n127 = call <vilib>:"Spark MAX Set Motor Type.vi"("error in (no error)"=w43, "Motor Type"=Spark_MAX_Motor_Type."Brushless", "MotorControlDevRef"=w44) -> ("error out"=w99:errorcluster, "MotorControlDeviceRef"=w100:T24)  [unwired: 7 in]
  n128 = call <vilib>:"CTRE_Phoenix_MotorControl_RefNumRegistrySet.vi"("error in (no error)"=w133, "refnum name"=w131, "PhoenixMotorControlDevRef"=w132) -> ()  [unwired: 7 in, 2 out]
  n129 = global read "Climb_Globals.vi" "Climb_Pivot"() -> (w139:string)
  n130 = call <vilib>:"CTRE_Phoenix_MotorControl_RefNumRegistrySet.vi"("error in (no error)"=w117, "refnum name"=w115, "PhoenixMotorControlDevRef"=w116) -> ()  [unwired: 7 in, 2 out]
  n131 = call <vilib>:"Spark MAX Set Idle Mode.vi"("error in (no error)"=w75, "Idle Mode"=Spark_MAX_Idle_Mode."Brake", "MotorControlDeviceRef in"=w72) -> ("error out"=w74:errorcluster, "MotorControlDeviceRef out"=w73:T24)  [unwired: 7 in]
  n132 = call <vilib>:"Spark MAX Set Output Advanced.vi"("error in (no error)"=w79, "Control Mode"=Spark_MAX_Control_Type."Percent VBus", "Setpoint"=0.0, "MotorControlDevRef"=w78) -> ("error out"=w156:errorcluster, "MotorControlDevRef"=w161:T24)  [unwired: 6 in]
  n133 = global read "Magazine_Globals.vi" "Magazine"() -> (w157:string)
  n134 = call <vilib>:"Spark MAX Set Idle Mode.vi"("error in (no error)"=w99, "Idle Mode"=Spark_MAX_Idle_Mode."Brake", "MotorControlDeviceRef in"=w100) -> ("error out"=w98:errorcluster, "MotorControlDeviceRef out"=w97:T24)  [unwired: 7 in]
  n135 = global read "Climb_Globals.vi" "Climb_Transverse"() -> (w130:string)
  n136 = global read "Turret_Globals.vi" "Turret_Spin"() -> (w218:string)
  n137 = call <vilib>:"Spark MAX Set Output Advanced.vi"("error in (no error)"=w74, "Control Mode"=Spark_MAX_Control_Type."Percent VBus", "Setpoint"=0.0, "MotorControlDevRef"=w73) -> ("error out"=w94:errorcluster, "MotorControlDevRef"=w141:T24)  [unwired: 6 in]
  n138 = call <vilib>:"Spark MAX Set PIDF Constants.vi"("error in"=w156, "PID Constants"=T6 {"P Gain"=0.0001, "I Gain"=0.0, "D Gain"=0.0, "F Gain"=0.5, "I Zone"=0.0, "Min Output"=-1.0, "Max Output"=1.0}, "MotorControlDeviceRef"=w161) -> ("error out"=w155:errorcluster, "MotorControlDeviceRef"=w162:T24)  [unwired: 7 in]
  n139 = call <vilib>:"CTRE_Phoenix_MotorControl_RefNumRegistrySet.vi"("error in (no error)"=w128, "refnum name"=w130, "PhoenixMotorControlDevRef"=w129) -> ()  [unwired: 7 in, 2 out]
  n140 = call <vilib>:"Spark MAX Set Output Advanced.vi"("error in (no error)"=w98, "Control Mode"=Spark_MAX_Control_Type."Percent VBus", "Setpoint"=0.0, "MotorControlDevRef"=w97) -> ("error out"=w195:errorcluster, "MotorControlDevRef"=w219:T24)  [unwired: 6 in]
  n141 = call <vilib>:"WPI_MotorControlRefNum Registry Set.vi"("error in (no error)"=w94, "refnum name"=w139, "MotorControlDevRef"=w141) -> ()  [unwired: 7 in, 2 out]
  n142 = call <vilib>:"WPI_MotorControlRefNum Registry Set.vi"("error in (no error)"=w155, "refnum name"=w157, "MotorControlDevRef"=w162) -> ()  [unwired: 7 in, 2 out]
  n143 = call <vilib>:"WPI_MotorControlRefNum Registry Set.vi"("error in (no error)"=w195, "refnum name"=w218, "MotorControlDevRef"=w219) -> ()  [unwired: 7 in, 2 out]
  "error out" <- "error in"
